vi "Vision Tracking X.vi"(0 "Tweak":dbl) -> (1 "right speed":dbl, 2 "left speed":dbl)   [LabVIEW 2013]
uses:
  typedefs/fg_typedef.ctl
  typedefs/vision data.ctl
  <vilib>/Rock Robotics/WPI/Camera/WPI_CameraImageSize.ctl
  <vilib>/addons/control/pid/pid.llb/PID (DBL).vi
  <vilib>/addons/control/pid/NI_PID_pid.lvlib
panel:
  out "R Rate":dbl
  out "R Distance":dbl
  out "L Rate":dbl
  out "L Distance":dbl
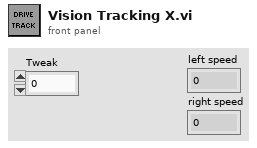
[diagram p1: front panel]
types:
  T1 = typedef "vision data.ctl" = cluster{"x":dbl, "y":dbl, "area":dbl, "width":dbl, "height":dbl, "Hot Goal Present?":bool, "distance":dbl}
  T2 = cluster{"proportional gain (Kc)":dbl, "integral time (Ti, min)":dbl, "derivative time (Td, min)":dbl}
  T3 = typedef "fg_typedef.ctl" = enum16{"Get", "Set"}
  T4 = typedef "WPI_EncoderDevRef.ctl" = cluster{"DevStatus":errorcluster, "EncoderIndex":T5, "CounterIndex":T6, "DistancePerCount":dbl, "Decoding Type":T7}
  T5 = typedef "FPGA_EncoderIdx.ctl" = enum8{"Enc 0", "Enc 1", "Enc 2", "Enc 3", "Invalid"}
  T6 = typedef "FPGA_CounterCtrSystemIndex.ctl" = enum8{"Ctr 0", "Ctr 1", "Ctr 2", "Ctr 3", "Ctr 4", "Ctr 5", "Ctr 6", "Ctr 7", "Invalid"}
  T7 = typedef "WPI_EncoderType.ctl" = enum16{"1x", "2x", "4x"}
  T8 = cluster{"x":bool, "y":bool, "area":bool, "width":bool, "height":bool, "Hot Goal Present?":bool, "distance":bool}
  T9 = typedef "WPI_CameraImageSize.ctl" = enum16{"640x480", "320x240", "160x120"}
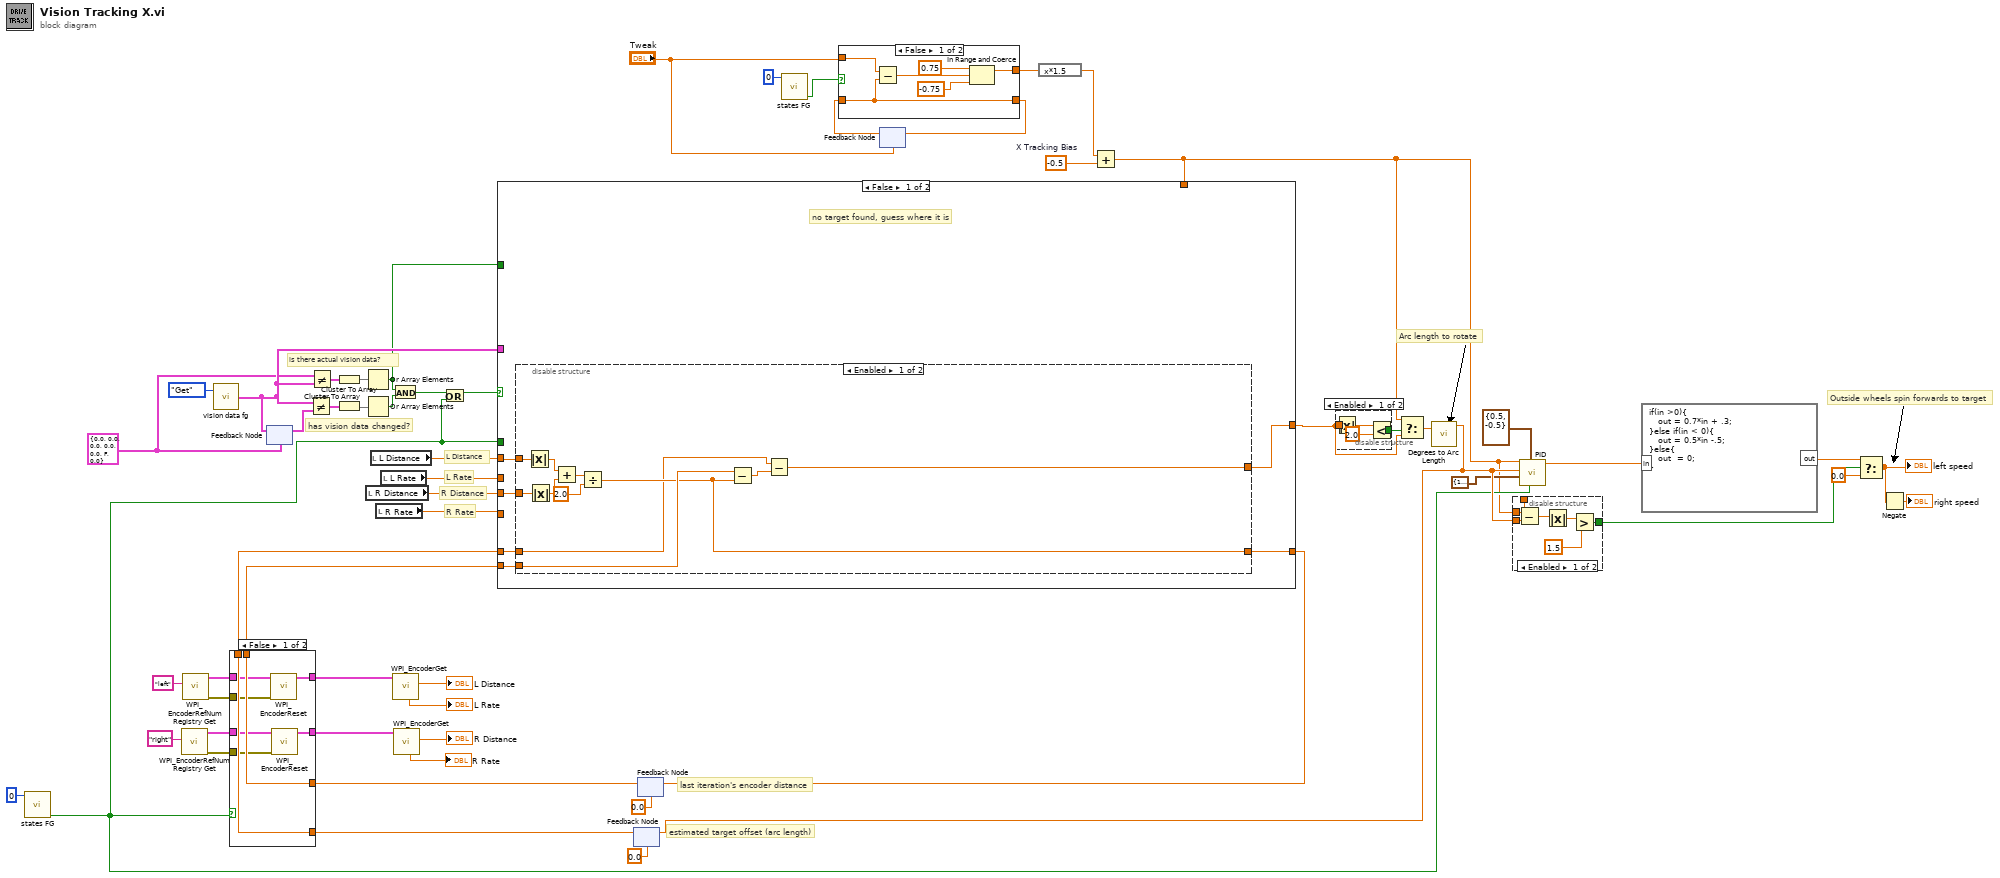
[diagram p0: block diagram]
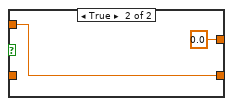
[diagram p2: hidden frame]
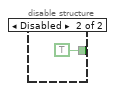
[diagram p3: hidden frame]
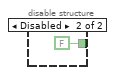
[diagram p4: hidden frame]
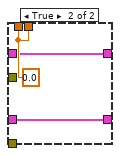
[diagram p5: hidden frame]
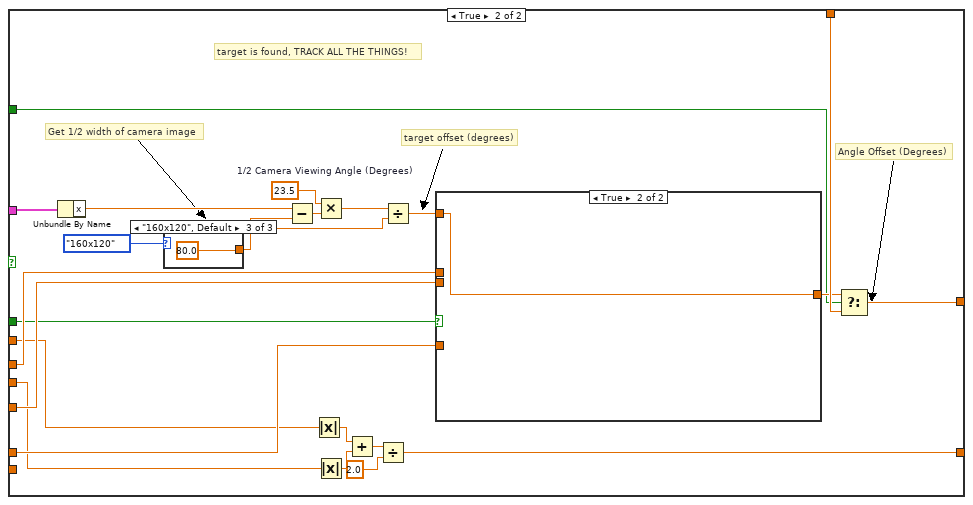
[diagram p7: hidden frame]
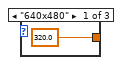
[diagram p8: hidden frame]
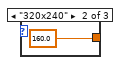
[diagram p9: hidden frame]
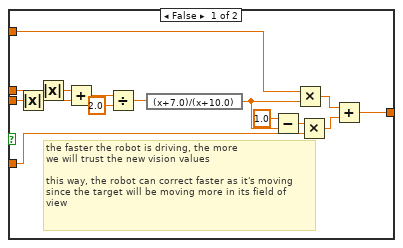
[diagram p10: hidden frame]
diagram:
  w1 = T1 {"x"=0.0, "y"=0.0, "area"=0.0, "width"=0.0, "height"=0.0, "Hot Goal Present?"=FALSE, "distance"=0.0} ("Output")
  w17 = -0.5  # X Tracking Bias
  # "Outside wheels spin forwards to target"
  # "Arc length to rotate"
  # "last iteration's encoder distance"
  # "R Rate"
  # "R Distance"
  # "L Rate"
  # "L Distance"
  # "estimated target offset (arc length)"
  # "has vision data changed?"
  # "is there actual vision data?"
  n1 = call "states FG.vi"("Loop ID"=0) -> ("first call?"=w14:bool)  [unwired: 7 in, 3 out]
  n2 = call <vilib>:"WPI_EncoderRefNum Registry Get.vi"("refnum name"="right") -> ("error out"=w36:errorcluster, "EncoderDevRef"=w37:T4)  [unwired: 9 in]
  n3 = call <vilib>:"WPI_EncoderRefNum Registry Get.vi"("refnum name"="left") -> ("error out"=w38:errorcluster, "EncoderDevRef"=w39:T4)  [unwired: 9 in]
  n4 = call "vision data fg.vi"("Menu"=fg_typedef."Get") -> ("Output"=w50:T1)  [unwired: 1 in]
  n5 = feedback-in #1(w50) -> ()
  n6 = feedback #1(w1) -> (w57:T1)
  n7 = Not Equal?(x=w50, y=w57) -> (x != y?=w52:T8)
  n8 = Not Equal?(x=w1, y=w50) -> (x != y?=w53:T8)
  n9 = Cluster To Array(cluster=w53) -> (array=w56:bool[])
  n10 = Cluster To Array(cluster=w52) -> (array=w55:bool[])
  n11 = Or Array Elements(Boolean array=w56) -> (logical OR=w24:bool)
  n12 = Or Array Elements(Boolean array=w55) -> (logical OR=w54:bool)
  n13 = local read "R Distance"() -> (w26:dbl)
  n14 = local read "L Distance"() -> (w28:dbl)
  n15 = local read "R Rate"() -> (w25:dbl)
  n16 = local read "L Rate"() -> (w27:dbl)
  n17 = And(x=w24, y=w54) -> (x .and. y?=w51:bool)
  n18 = Or(x=w51, y=w14) -> (x .or. y?=w46:bool)
  n19 = feedback #2(0.0) -> (w47:dbl)
  n20 = feedback #3(0.0) -> (w42:dbl)
  n21 = case shown="False" w14 {
    tunnel: w47 -> [w66 _]
    tunnel: [w66 w69] -> w45
    tunnel: [w65 w69] -> w43
    tunnel: w42 -> [w65 _]
    tunnel: w39 -> [w64 w68]
    tunnel: w38 -> [w63 _]
    tunnel: w37 -> [w62 w67]
    tunnel: w36 -> [w61 _]
    tunnel: [w60 w68] -> w35
    tunnel: [w59 w67] -> w34
    frame False {
      n22 = call <vilib>:"WPI_EncoderReset.vi"("error in (no error)"=w63, "EncoderDevRef"=w64) -> ("EncoderDevRef"=w60:T4)  [unwired: 8 in, 1 out]
      n23 = call <vilib>:"WPI_EncoderReset.vi"("error in (no error)"=w61, "EncoderDevRef"=w62) -> ("EncoderDevRef"=w59:T4)  [unwired: 8 in, 1 out]
    }
    frame True {
      w69 = 0.0
    }
  }
  n24 = call <vilib>:"WPI_EncoderGet.vi"("EncoderDevRef"=w35) -> ("Distance"=→"L Distance":dbl, "Rate"=→"L Rate":dbl)  [unwired: 5 in, 4 out]
  n25 = call <vilib>:"WPI_EncoderGet.vi"("EncoderDevRef"=w34) -> ("Distance"=→"R Distance":dbl, "Rate"=→"R Rate":dbl)  [unwired: 5 in, 4 out]
  n26 = call "states FG.vi"("Loop ID"=0) -> ("first call?"=w8:bool)  [unwired: 7 in, 3 out]
  n27 = feedback #4("Tweak") -> (w7:dbl)
  n28 = case shown="False" w8 {
    tunnel: "Tweak" -> [w75 w77]
    tunnel: [w74 w77] -> w5
    tunnel: w7 -> [w74 _]
    tunnel: [w71 0.0 ("upper limit")] -> w3
    frame False {
      n29 = Subtract(x=w75, y=w74) -> (x-y=w70:dbl)
      n30 = In Range and Coerce(upper limit=0.75, x=w70, lower limit=-0.75) -> (coerced(x)=w71:dbl)  [unwired: 1 out]
    }
    frame True {
    }
  }
  n31 = feedback-in #4(w5) -> ()
  n32 = expression code="x*1.5"(w3) -> (w2:dbl)
  n33 = Add(x=w2, y=w17) -> (x+y=w4:dbl)
  n34 = case shown="False" w46 {
    tunnel: w50 -> [_ w117]
    tunnel: w27 -> [_ w107]
    tunnel: w28 -> [w83 w101]
    tunnel: w26 -> [w82 w100]
    tunnel: w25 -> [_ w106]
    tunnel: [w78 w96] -> w12
    tunnel: w45 -> [w79 w116]
    tunnel: w4 -> [_ w109]
    tunnel: w43 -> [w81 _]
    tunnel: [w80 w99] -> w33
    tunnel: w14 -> [_ w98]
    tunnel: w24 -> [_ w97]
    frame False {
      # "no target found, guess where it is"
      n35 = disable-structure shown="Enabled" {
        disable-tunnel: w83 -> [w94 _]
        disable-tunnel: w82 -> [w93 _]
        disable-tunnel: w81 -> [w88 _]
        disable-tunnel: [w87 _] -> w80
        disable-tunnel: w79 -> [w85 _]
        disable-tunnel: [w84 _] -> w78
        frame Enabled {
          n36 = Absolute Value(x=w94) -> (abs(x)=w92:dbl)
          n37 = Absolute Value(x=w93) -> (abs(x)=w91:dbl)
          n38 = Add(x=w92, y=w91) -> (x+y=w90:dbl)
          n39 = Divide(x=w90, y=2.0) -> (x/y=w87:dbl)
          n40 = Subtract(x=w88, y=w87) -> (x-y=w86:dbl)
          n41 = Subtract(x=w85, y=w86) -> (x-y=w84:dbl)
        }
        frame Disabled {
        }
      }
    }
    frame True {
      w113 = 23.5  # 1/2 Camera Viewing Angle (Degrees)
      # "Angle Offset (Degrees)"
      # "target offset (degrees)"
      # "Get 1/2 width of camera image"
      # "target is found, TRACK ALL THE THINGS!"
      n42 = Unbundle By Name(w117) -> ("x"=w115:dbl)
      n43 = case shown="\"160x120\", Default" WPI_CameraImageSize."160x120" ("Image Size") {
        tunnel: [320.0 160.0 80.0] -> w110
        frame "640x480" {
        }
        frame "320x240" {
        }
        frame "160x120", Default {
        }
      }
      n44 = Subtract(x=w115, y=w110) -> (x-y=w114:dbl)
      n45 = Absolute Value(x=w101) -> (abs(x)=w102:dbl)
      n46 = Multiply(x=w113, y=w114) -> (x*y=w112:dbl)
      n47 = Absolute Value(x=w100) -> (abs(x)=w103:dbl)
      n48 = Add(x=w102, y=w103) -> (x+y=w104:dbl)
      n49 = Divide(x=w104, y=2.0) -> (x/y=w99:dbl)
      n50 = Divide(x=w112, y=w110) -> (x/y=w111:dbl)
      n51 = case shown="True" w98 {
        tunnel: w107 -> [w131 _]
        tunnel: w106 -> [w130 _]
        tunnel: w111 -> [w123 w136]
        tunnel: [w122 w136] -> w108
        tunnel: w116 -> [w121 _]
        frame False {
          # "the faster the robot is driving, the more\nwe will trust the new vision values\n\nthis way, the robot can correct faster as it's moving\nsince the target will be moving more in its field of\nview"
          n52 = Absolute Value(x=w130) -> (abs(x)=w135:dbl)
          n53 = Absolute Value(x=w131) -> (abs(x)=w134:dbl)
          n54 = Add(x=w134, y=w135) -> (x+y=w132:dbl)
          n55 = Divide(x=w132, y=2.0) -> (x/y=w129:dbl)
          n56 = expression code="(x+7.0)/(x+10.0)"(w129) -> (w124:dbl)
          n57 = Subtract(x=1.0, y=w124) -> (x-y=w127:dbl)
          n58 = Multiply(x=w123, y=w124) -> (x*y=w125:dbl)
          n59 = Multiply(x=w127, y=w121) -> (x*y=w126:dbl)
          n60 = Add(x=w125, y=w126) -> (x+y=w122:dbl)
        }
        frame True {
        }
      }
      n61 = Select(t=w108, s=w97, f=w109) -> (s? t:f=w96:dbl)
    }
  }
  n62 = feedback-in #3(w33) -> ()
  n63 = disable-structure shown="Enabled" {
    disable-tunnel: [w139 FALSE] -> w21
    disable-tunnel: w12 -> [w137 _]
    frame Enabled {
      n64 = Absolute Value(x=w137) -> (abs(x)=w138:dbl)
      n65 = Less?(x=w138, y=2.0) -> (x < y?=w139:bool)
    }
    frame Disabled {
    }
  }
  n66 = Select(t=w4, s=w21, f=w12) -> (s? t:f=w22:dbl)
  n67 = call "Degrees to Arc Length.vi"("Angle"=w22) -> ("Arc Length (inches)"=w16:dbl)  [unwired: 4 in]
  n68 = feedback-in #2(w16) -> ()
  n69 = disable-structure shown="Enabled" {
    disable-tunnel: w4 -> [w142 _]
    disable-tunnel: w16 -> [w146 _]
    disable-tunnel: [w143 TRUE] -> w19
    disable-tunnel: [w142 _] -> _
    frame Enabled {
      n70 = Subtract(x=w142, y=w146) -> (x-y=w147:dbl)
      n71 = Absolute Value(x=w147) -> (abs(x)=w145:dbl)
      n72 = Greater?(x=w145, y=1.5) -> (0:w143:bool)
    }
    frame Disabled {
    }
  }
  n73 = call-poly <vilib>:"PID.vi"("reinitialize? (F)"=w14, "output range"=cluster{"output high":dbl, "output low":dbl} {"output high"=0.5, "output low"=-0.5}, "PID gains"=T2 {"proportional gain (Kc)"=1.0, "integral time (Ti, min)"=0.01, "derivative time (Td, min)"=0.0}, "process variable"=w16, "setpoint"=w4) -> ("output"=w11:dbl)  [unwired: 5 in, 1 out]
  n74 = formula code="if(in >0){\n   out = 0.7*in + .3;\n}else if(in < 0){\n   out = 0.5*in -.5;\n}else{\n   out  = 0;\n}"("in"=w11) -> ("out"=w10:dbl)
  n75 = Select(t=w10, s=w19, f=0.0) -> (s? t:f=w20:dbl)
  "left speed" <- w20
  n76 = Negate(x=w20) -> (-x=→"right speed":dbl)
